vi "Test_Contactor.vi"(2 "cell sum":dbl, 4 "Limits":T2, 8 "error in (no error)":errorcluster, 11 "connection ID":refnum<k5>) -> (0 "error out":errorcluster, 1 "cont open reply":string, 3 "connection ID out":refnum<k5>, 7 "results":T1[](array[typedef]))   [LabVIEW 2026]
uses:
  Limits.ctl
  Result.ctl
  Test_Contactor.ctl
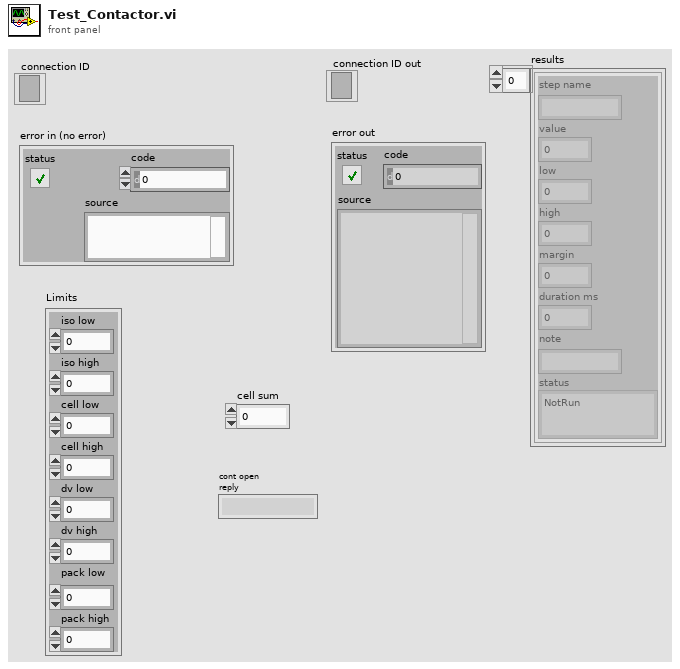
[diagram p1: front panel]
types:
  T1 = typedef "Result.ctl" = cluster{"step name":string, "value":dbl, "low":dbl, "high ":dbl, "margin":dbl, "duration ms":dbl, "note":string, "status":enum16{"NotRun", "Pass", "Fail", "Skipped"}}
  T2 = typedef "Limits.ctl" = cluster{"iso low":dbl, "iso high":dbl, "cell low":dbl, "cell high":dbl, "dv low":dbl, "dv high":dbl, "pack low":dbl, "pack high":dbl}
  T3 = typedef "Test_Contactor.ctl" = enum16{"NotRun", "Pass", "Fail", "Skipped"}
  T4 = cluster{"step name":string, "value":dbl, "low":dbl, "high ":dbl, "margin":dbl, "duration ms":dbl, "note":string, "status":enum16{"NotRun", "Pass", "Fail", "Skipped"}}
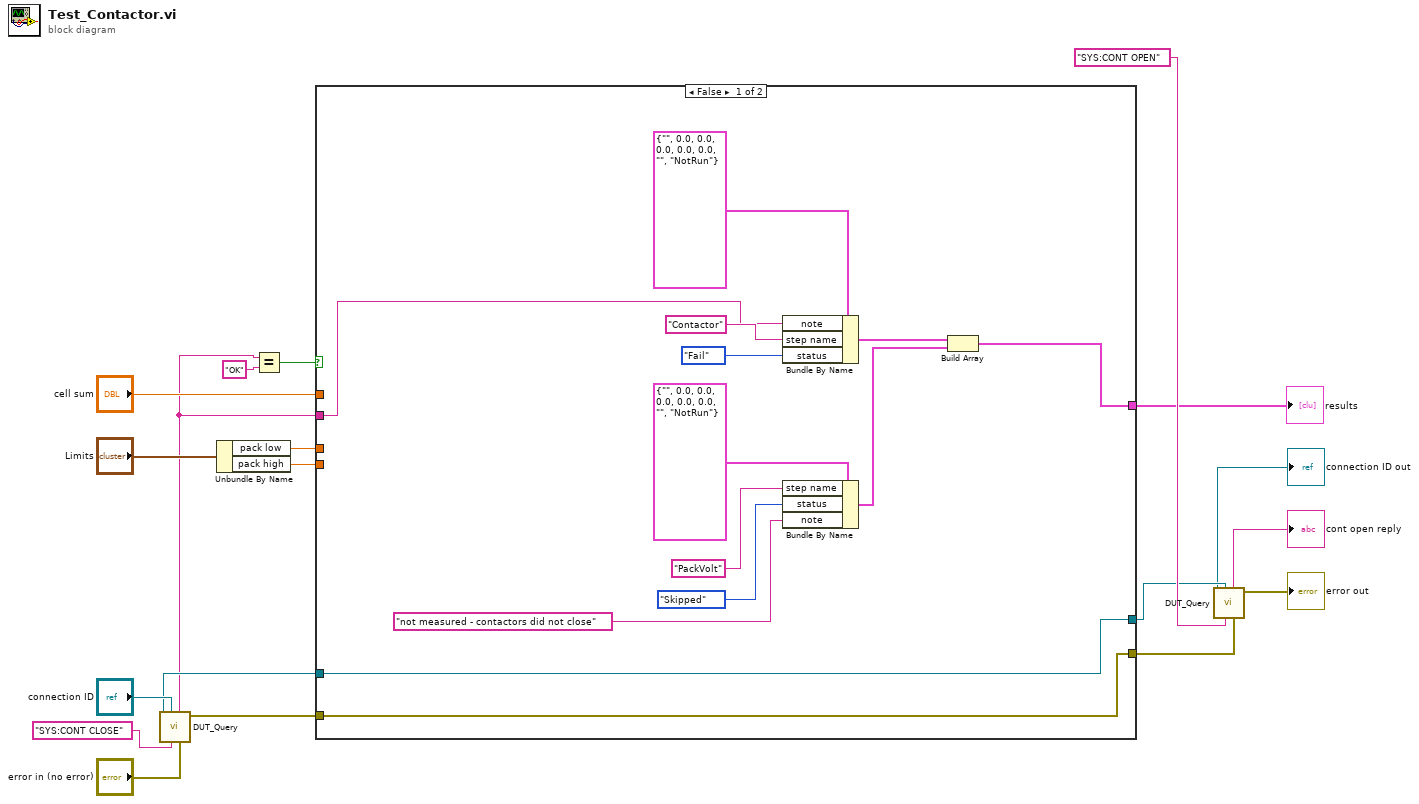
[diagram p0: block diagram]
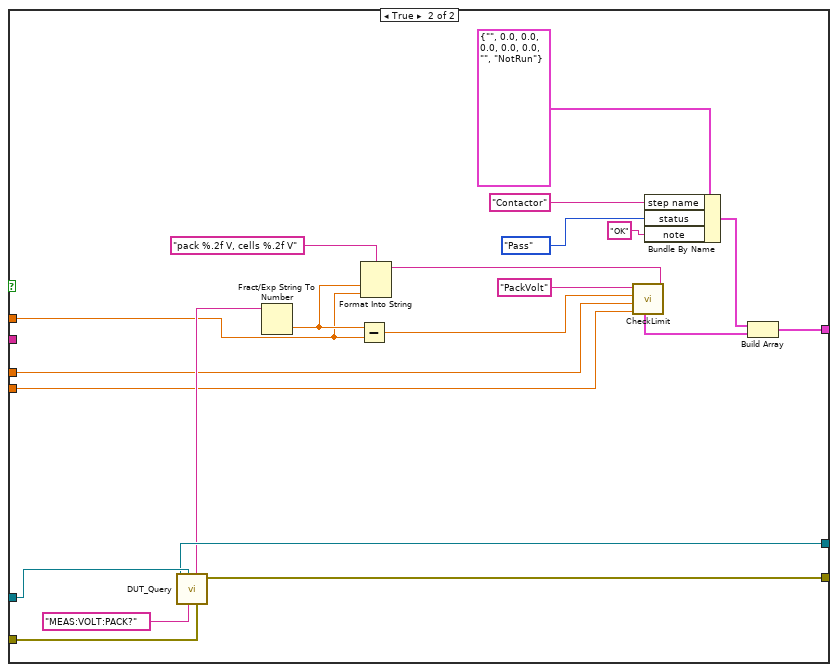
[diagram p2: hidden frame]
diagram:
  n1 = call "DUT_Query.vi"("error in (no error)"="error in (no error)", "command"="SYS:CONT CLOSE", "connection ID"="connection ID") -> ("error out"=w13:errorcluster, "reply"=w8:string, "connection ID out"=w14:refnum<k5>)  [unwired: 5 in, 1 out]
  n2 = Unbundle By Name("Limits") -> ("pack low"=w10:dbl, "pack high"=w9:dbl)
  n3 = Equal?(x=w8, y="OK") -> (x = y?=w15:bool)
  n4 = case shown="False" w15 {
    tunnel: w14 -> [w21 w52]
    tunnel: [w21 w51] -> w5
    tunnel: w13 -> [w20 w50]
    tunnel: [w20 w49] -> w4
    tunnel: "cell sum" -> [_ w41]
    tunnel: w10 -> [_ w47]
    tunnel: w9 -> [_ w46]
    tunnel: [w22 w33] -> w1
    tunnel: w8 -> [w25 _]
    frame False {
      n5 = Bundle By Name(cluster=T1 {"step name"="", "value"=0.0, "low"=0.0, "high "=0.0, "margin"=0.0, "duration ms"=0.0, "note"="", "status"=enum."NotRun"} ("Result"), "note"=w25, "step name"="Contactor", "status"=Test_Contactor."Fail") -> (w24:T1)
      n6 = Bundle By Name(cluster=T1 {"step name"="", "value"=0.0, "low"=0.0, "high "=0.0, "margin"=0.0, "duration ms"=0.0, "note"="", "status"=enum."NotRun"} ("Result"), "step name"="PackVolt", "status"=enum16{"NotRun", "Pass", "Fail", "Skipped"}."Skipped", "note"="not measured - contactors did not close") -> (w23:T1)
      n7 = Build Array(w24, w23) -> (w22:T1[])
    }
    frame True {
      n8 = call "DUT_Query.vi"("error in (no error)"=w50, "command"="MEAS:VOLT:PACK?", "connection ID"=w52) -> ("error out"=w49:errorcluster, "reply"=w48:string, "connection ID out"=w51:refnum<k5>)  [unwired: 5 in, 1 out]
      n9 = Fract/Exp String To Number(string=w48) -> (number=w42:dbl)  [unwired: 3 in, 1 out]
      n10 = Subtract(x=w42, y=w41) -> (x-y=w45:dbl)
      n11 = Format Into String(format string="pack %.2f V, cells %.2f V", w42, w41) -> (resulting string=w40:string)  [unwired: 2 in, 1 out]
      n12 = call "CheckLimit.vi"("note"=w40, "high"=w46, "low"=w47, "value"=w45, "step name"="PackVolt") -> ("Result"=w35:T4)  [unwired: 4 in, 2 out]
      n13 = Bundle By Name(cluster=T1 {"step name"="", "value"=0.0, "low"=0.0, "high "=0.0, "margin"=0.0, "duration ms"=0.0, "note"="", "status"=enum."NotRun"} ("Result"), "step name"="Contactor", "status"=enum16{"NotRun", "Pass", "Fail", "Skipped"}."Pass", "note"="OK") -> (w34:T1)
      n14 = Build Array(w34, w35) -> (w33:T1[])
    }
  }
  "results" <- w1
  n15 = call "DUT_Query.vi"("error in (no error)"=w4, "command"="SYS:CONT OPEN", "connection ID"=w5) -> ("error out"=→"error out":errorcluster, "reply"=→"cont open reply":string, "connection ID out"=→"connection ID out":refnum<k5>)  [unwired: 5 in, 1 out]
